vi "Point Inside Bounds.vi"(10 "Point":T1, 11 "Bounds":T2) -> (3 "Inside?":bool)   [LabVIEW 2019, in "2D.lvlib"]
doc: "Test if a given point is inside the bounding rectangle. Returns true if the point is within the bounds, false otherwise."
uses:
  <vilib>/Utility/miscctls.llb/LVRectTypeDef.ctl
  Point.ctl
  2D.lvlib
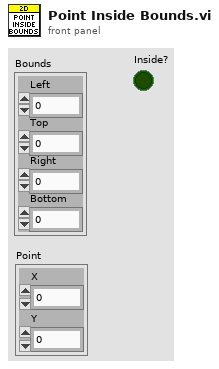
[diagram p1: front panel]
types:
  T1 = typedef "2D.lvlib/Point.ctl" = cluster{"X":i16, "Y":i16}
  T2 = typedef "LVRectTypeDef.ctl" = cluster{"Left":i16, "Top":i16, "Right":i16, "Bottom":i16}
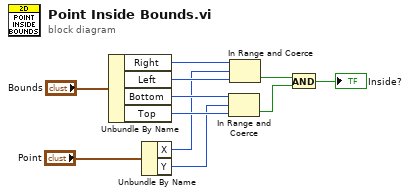
[diagram p0: block diagram]
diagram:
  n1 = Unbundle By Name("Bounds") -> ("Right"=w10:i16, "Left"=w9:i16, "Bottom"=w8:i16, "Top"=w7:i16)
  n2 = Unbundle By Name("Point") -> ("X"=w5:i16, "Y"=w4:i16)
  n3 = In Range and Coerce(upper limit=w8, x=w4, lower limit=w7) -> (In Range?=w2:bool)  [unwired: 1 out]
  n4 = In Range and Coerce(upper limit=w10, x=w5, lower limit=w9) -> (In Range?=w3:bool)  [unwired: 1 out]
  n5 = And(x=w3, y=w2) -> (x .and. y?=→"Inside?":bool)
